vi "all_stages.vi"() -> ()   [LabVIEW 2024]
uses:
  O:/DSG/Tyler/EIC/DIRC/daq/automated/Thorlabs.MotionControl.Controls.dll
  Thorlabs.MotionControl.Controls.dll
  O:/DSG/Tyler/EIC/DIRC/daq/automated/Thorlabs.MotionControl.IntegratedStepperMotorsCLI.dll
  Thorlabs.MotionControl.IntegratedStepperMotorsCLI.dll
  O:/DSG/Tyler/EIC/DIRC/daq/automated/Thorlabs.MotionControl.Benchtop.StepperMotorCLI.dll
  Thorlabs.MotionControl.Benchtop.StepperMotorCLI.dll
  <instrlib>/Keithley 6517/Keithley 6517.lvlib
panel:
  out "ySeq_hist":dbl[][](array[numeric])
  out "xSeq_hist":dbl[][](array[numeric])
  out "xSeq_diff":dbl[](array[numeric])
  out "ySeq_diff":dbl[](array[numeric])
  out "ySeq_in":dbl[](array[numeric])
  out "xSeq_in":dbl[](array[numeric])
  out "ySeq_res":dbl[](array[numeric])
  out "xSeq_res":dbl[](array[numeric])
  in  "go_seq_test":bool
  out "PD Values":cluster{"PD1":dbl, "PD2":dbl, "PD3":dbl}
  out "last-PD":dbl[](array[numeric])=[1.0, 1.0, 1.0]
  in  "move-bar":bool
  in  "mode-select":enum32{"IR", "Pure", "Bulk", "Bar Out"}(radio) caption="Mode Select"
  in  "auto-align-grid":bool
  in  "auto-delta":dbl=0.5
  out "max value":dbl
  out "xOut":dbl
  out "yOut":dbl
  out "max indexes":i32[](array[numeric])
  in  "k":dbl=25.0
  in  "N trials":dbl=16.0
  in  "auto-align":bool
  out "pd_angle":dbl
  out "brewster_angle":dbl
  out "meter-visa":refnum<visa-resource-name>
  out "loop-rate":u32
  out "meter-stat":bool caption="Log Status"
  out "file-stat":bool caption="Log Status"
  out "stage-stat":bool caption="Log Status"
  out "last-save-time":string caption="Time of Last Save:"
  out "pd_y_pos":dbl
  out "pd_x_pos":dbl
  out "bar_y_pos":dbl
  out "bar_x_pos":dbl
  in  "nSamples":dbl=50.0 caption="# Samples"
  out "Current Time:":string
  in  "save-data":bool
  in  "bar-note":bool
  out "pd3_v":dbl caption="PD 3" format="%#.4g"
  out "pd2_v":dbl caption="PD 2" format="%#.4g"
  out "pd1_v":dbl caption="PD 1" format="%#.4g"
  out "meter-error":errorcluster
  out "log-error":errorcluster
  out "log-path":path caption="Path Data Will Save To:"
  out "start-msg":string
  out "stage-error":errorcluster
  in  "PD Angle":refnum<k24>(container)
  in  "Brewster":refnum<k24>(container)
  in  "PD Y":refnum<k24>(container)
  in  "PD X":refnum<k24>(container)
  in  "BAR Y":refnum<k24>(container)
  in  "stop":bool
  in  "BAR X":refnum<k24>(container)
  out "pd-plt":cluster{"[0]":dbl, "[1]":dbl, "[2]":dbl}(graph) caption="Measurement History"
  # "EXPERT DEBUGGING INFO"
  # "A"
  # "A"
  # "A"
  # "Work In Progress - please do not use"
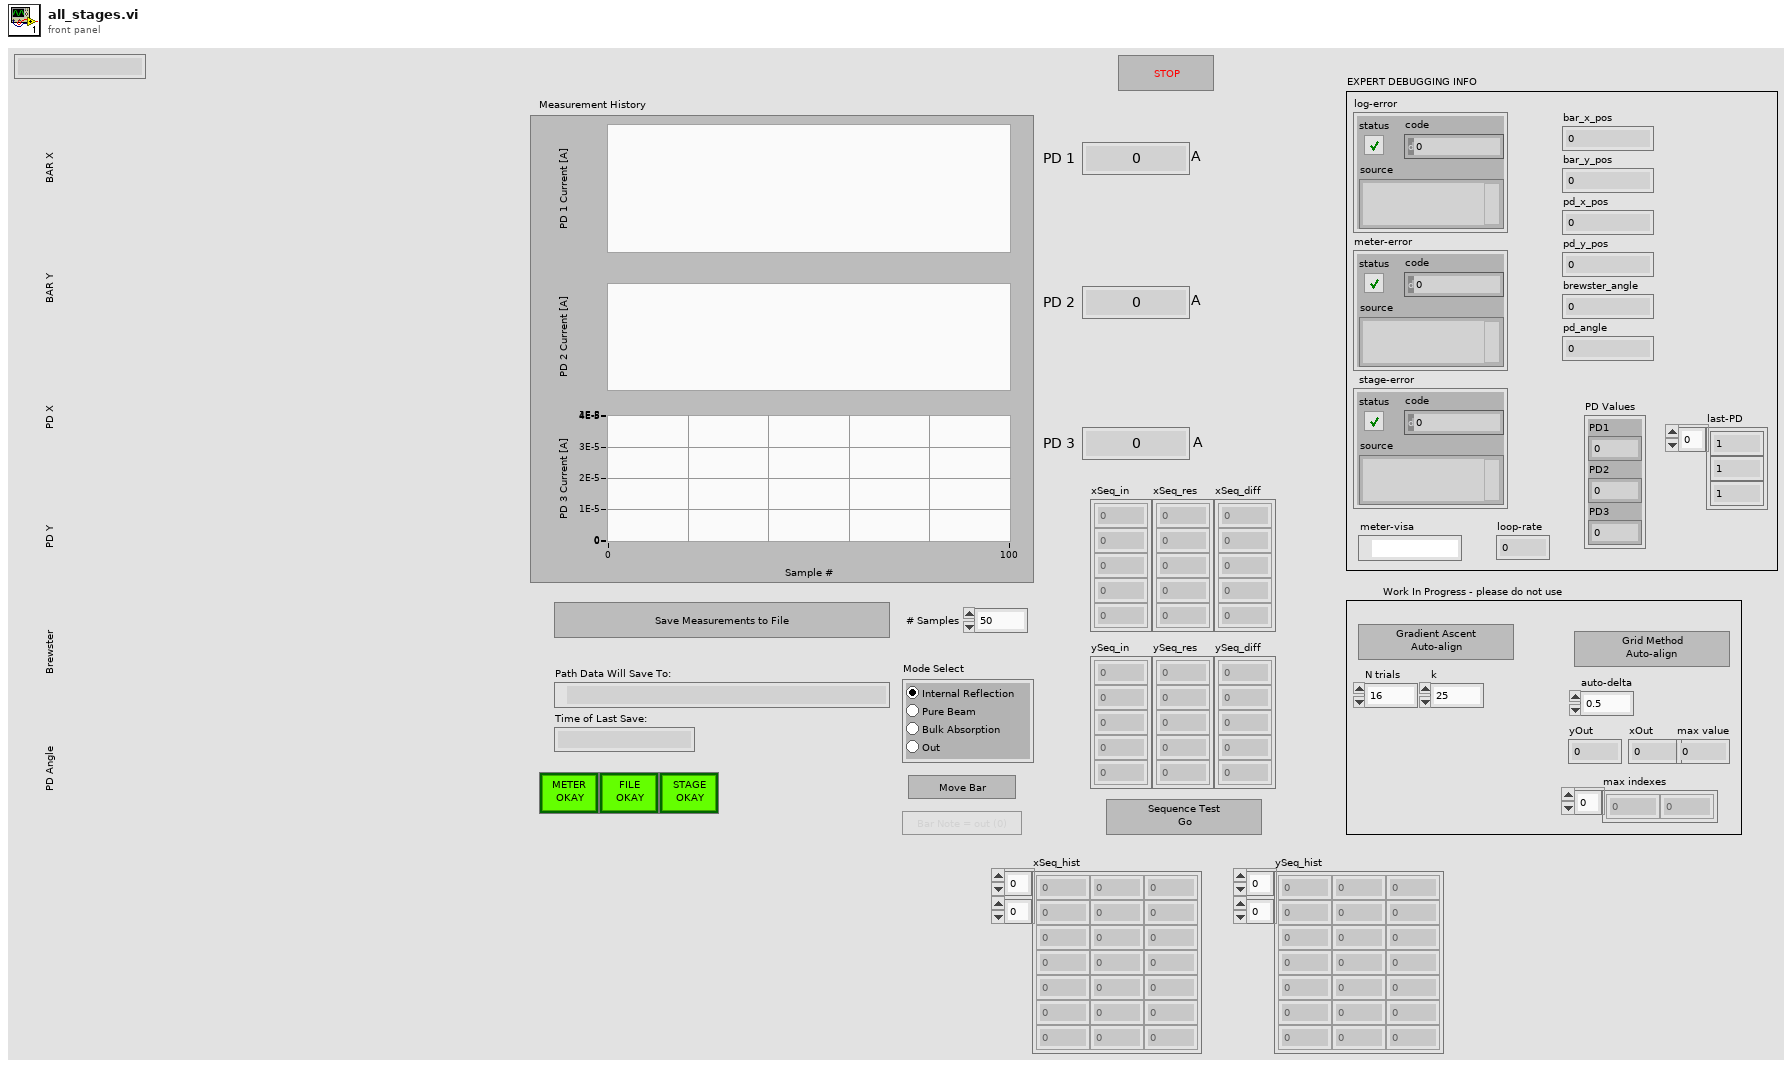
[diagram p1: front panel]
types:
  T1 = cluster{"Bar X":refnum<k24>, "Bar Y":refnum<k24>, "PD X":refnum<k24>, "PD Y":refnum<k24>, "Brewster":refnum<k24>, "PD Angle":refnum<k24>}
  T2 = enum16{"open", "replace", "create", "open or create", "replace or create", "replace or create with confirmation"}
  T3 = cluster{"error":bool, "code":i32, "source":string}
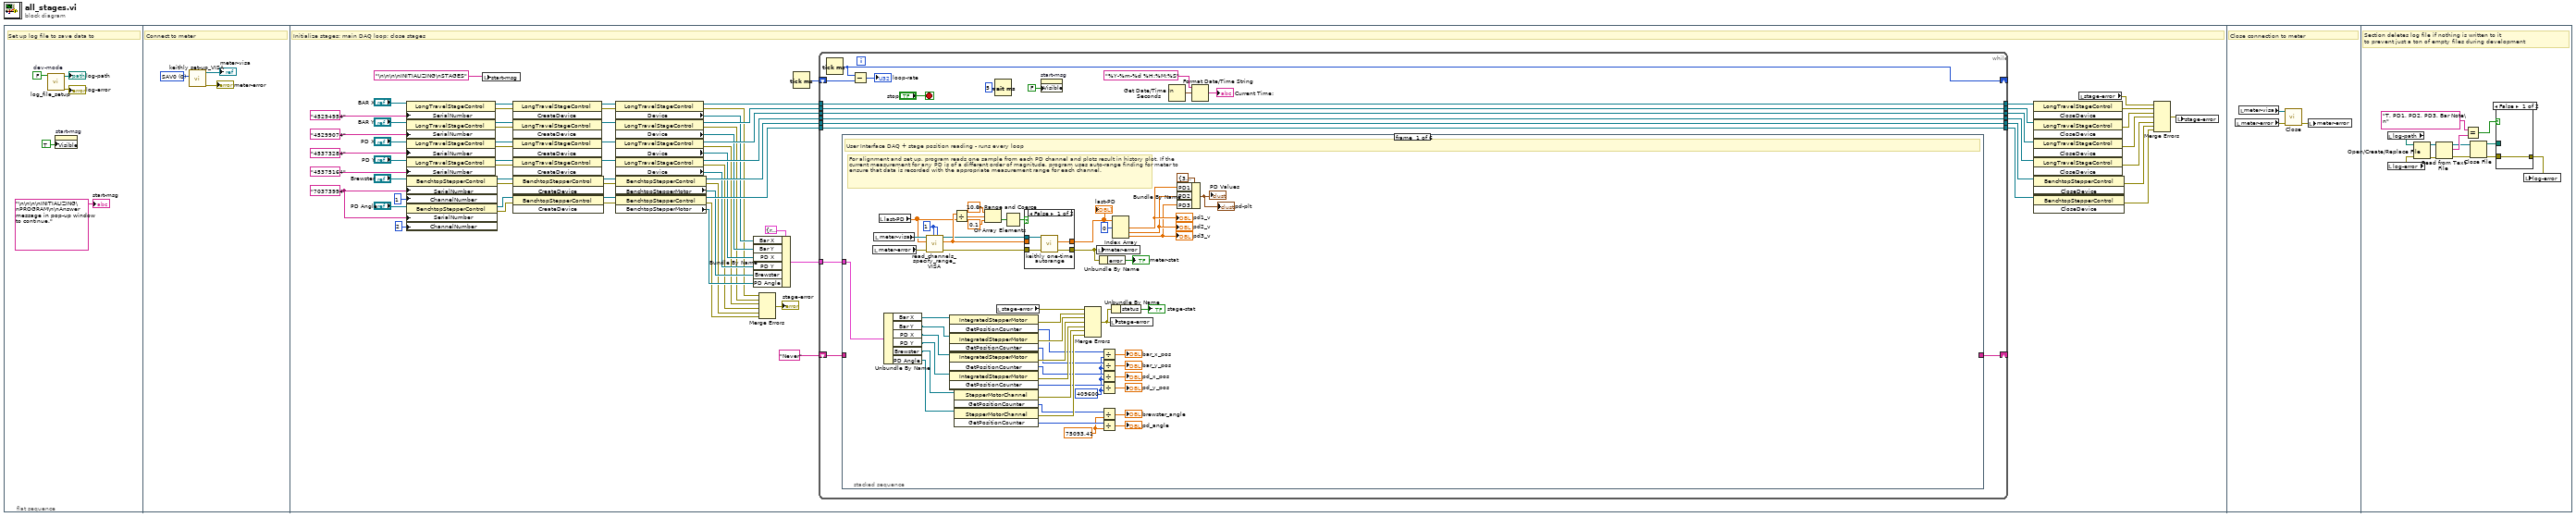
[diagram p0: block diagram]
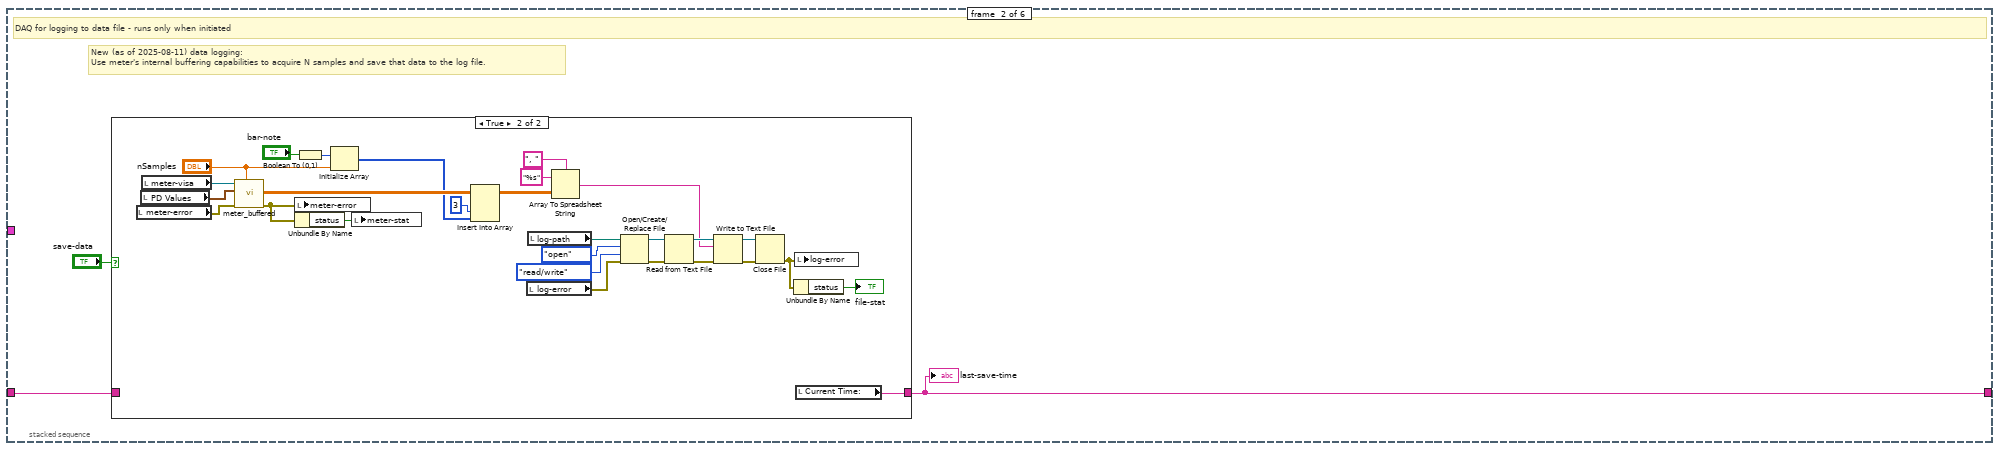
[diagram p3: hidden frame]
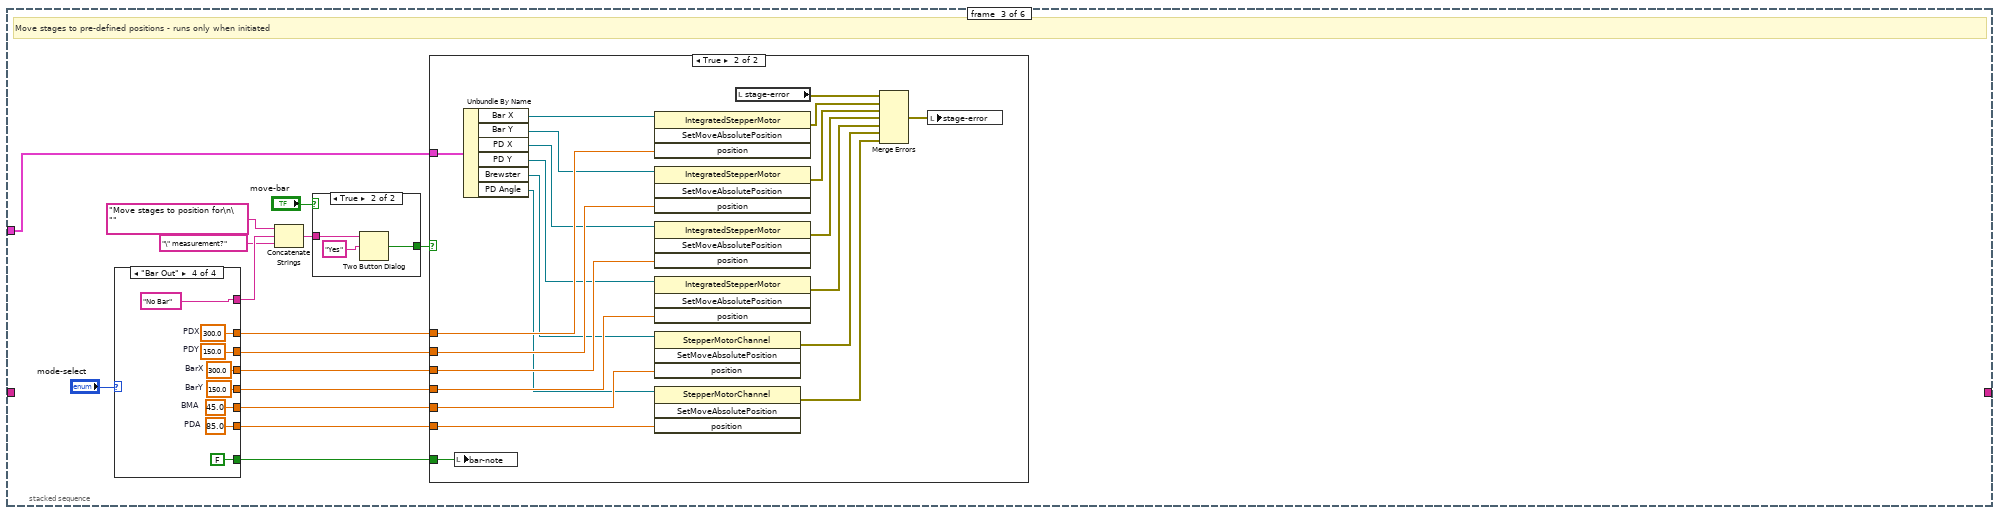
[diagram p5: hidden frame]
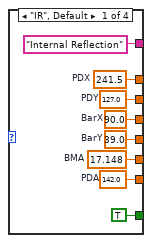
[diagram p7: hidden frame]
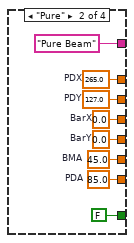
[diagram p8: hidden frame]
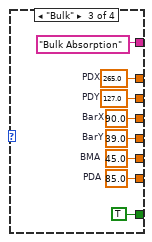
[diagram p9: hidden frame]
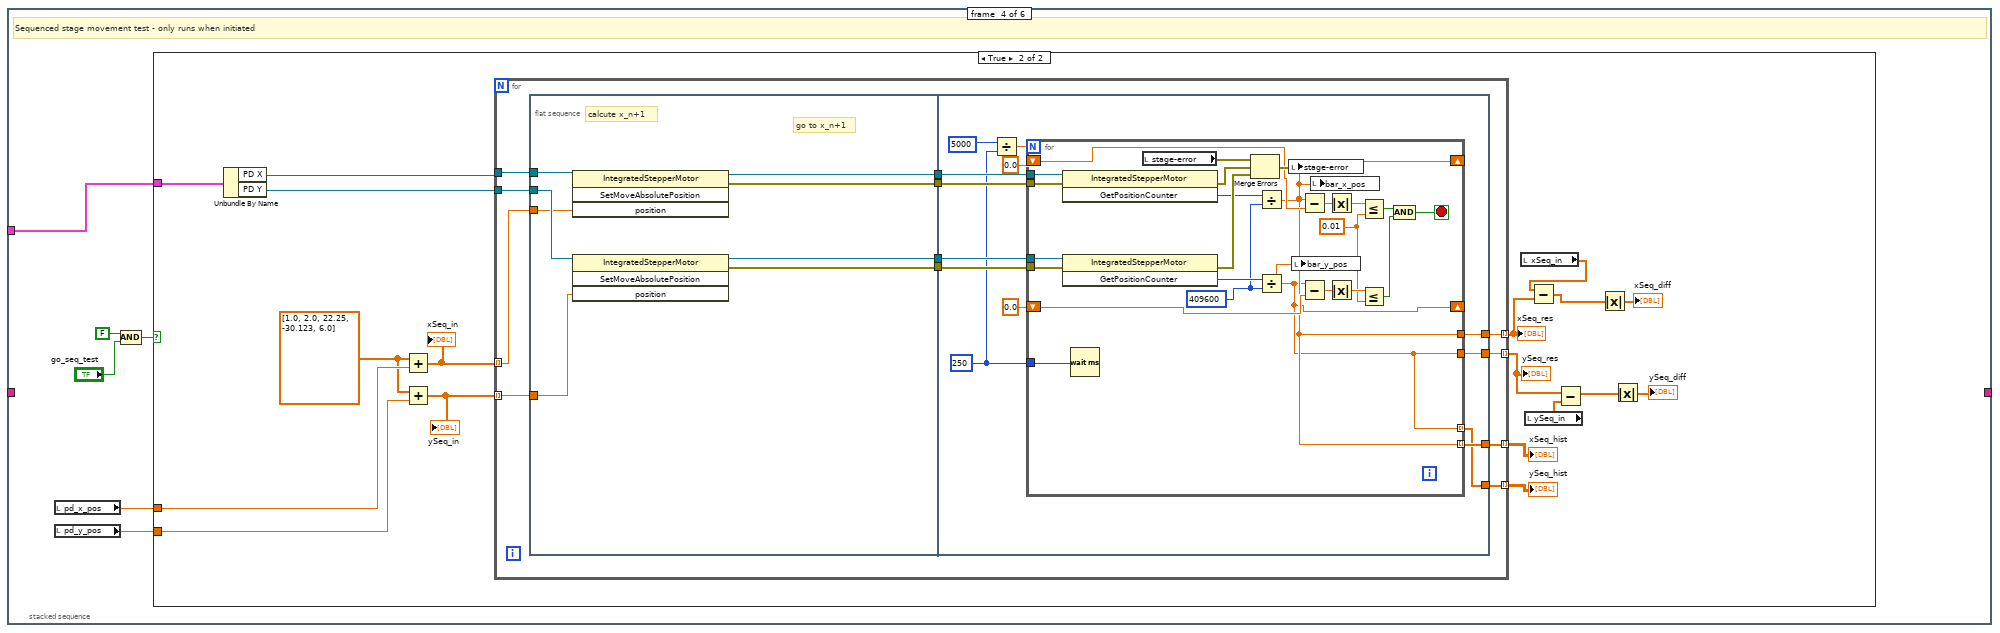
[diagram p11: hidden frame]
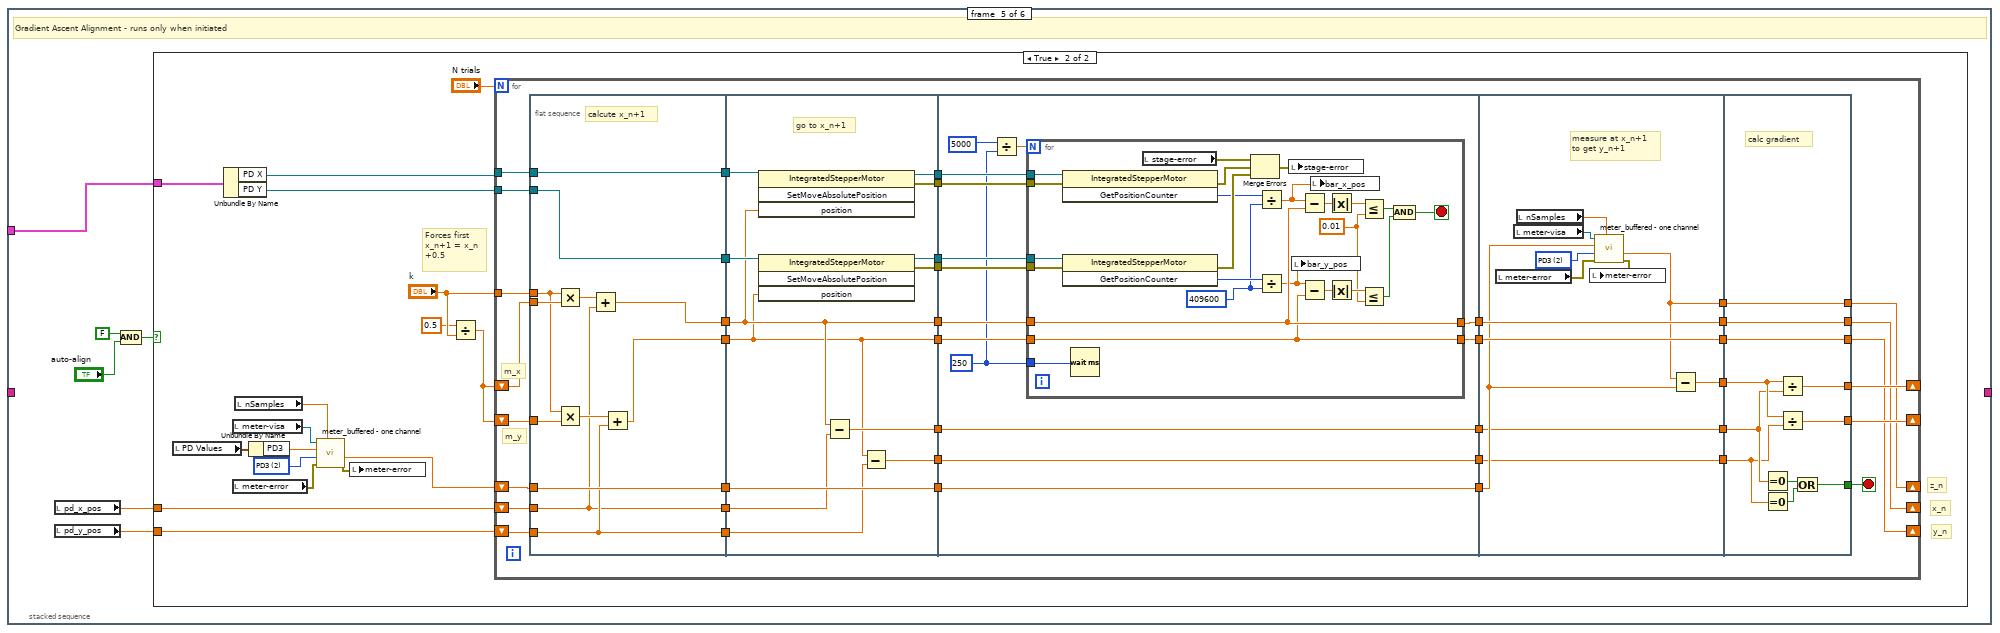
[diagram p13: hidden frame]
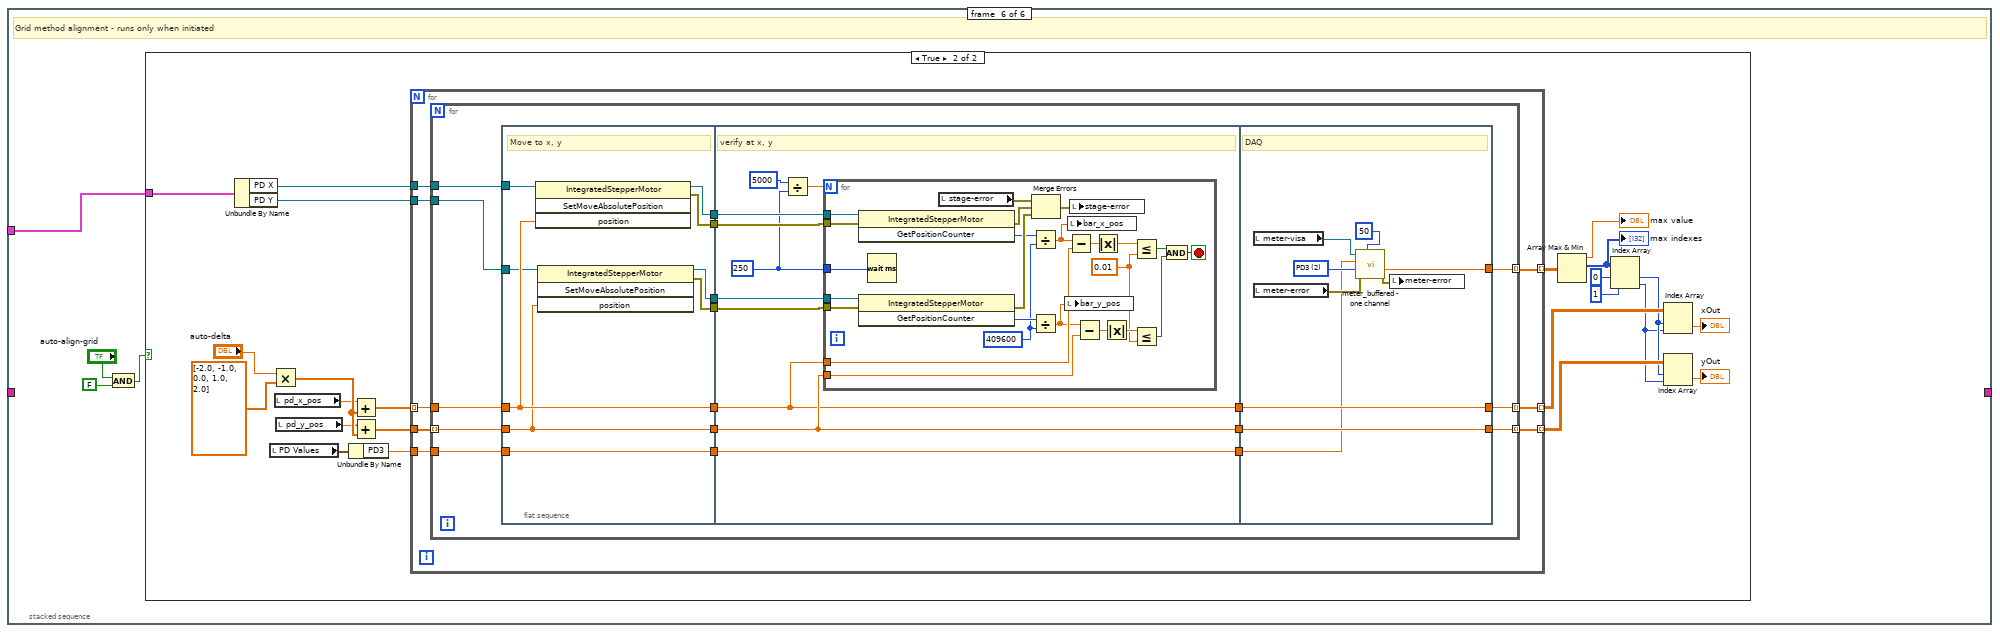
[diagram p15: hidden frame]
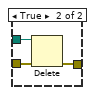
[diagram p17: hidden frame]
diagram:
  n1 = flat-sequence {
    frame #0 {
      w5 = FALSE  # dev-mode
      # "Set up log file to save data to"
      n2 = call "log_file_setup.vi"("dev-mode"=w5) -> ("error out"=→"log-error":errorcluster, "appended path"=→"log-path":path)  [unwired: 8 in, 1 out]
      n3 = property on="start-msg" class="Str"("Visible"=TRUE) -> ()  [unwired: 2 in, 2 out]
      "start-msg" <- "\n\n\n\nINITIALIZING\nPROGRAM\n\nAnswer message in pop-up window to continue." ("String")
    }
    frame #1 {
      w6 = i16 0 items=["SAV0", "SAV1", "SAV2", "SAV3", "SAV4", "SAV5", "SAV6", "SAV7", "SAV8", "SAV9", "RST", "Preset"] ("ConfigOpt")
      # "Connect to meter"
      n4 = call "keithly set-up_VISA.vi"("ConfigOpt"=w6) -> ("error out"=→"meter-error":errorcluster, "meter-VISA"=→"meter-visa":refnum<visa-resource-name>)  [unwired: 9 in]
    }
    frame #2 {
      w57 = "70373994" ("SerialNumber")
      # "Initialize stages; main DAQ loop; close stages"
      n5 = property class="LongTravelStageControl"(reference="BAR X", "SerialNumber"="45294954") -> (reference out=w79:refnum<k24>, error out=w71:errorcluster)  [unwired: 1 in]
      n6 = property class="LongTravelStageControl"(reference="BAR Y", "SerialNumber"="45299074") -> (reference out=w77:refnum<k24>, error out=w70:errorcluster)  [unwired: 1 in]
      n7 = property class="LongTravelStageControl"(reference="PD X", "SerialNumber"="45373284") -> (reference out=w74:refnum<k24>, error out=w69:errorcluster)  [unwired: 1 in]
      n8 = property class="LongTravelStageControl"(reference="PD Y", "SerialNumber"="45375164") -> (reference out=w73:refnum<k24>, error out=w68:errorcluster)  [unwired: 1 in]
      n9 = property class="BenchtopStepperControl"(reference="Brewster", "SerialNumber"=w57, "ChannelNumber"=1) -> (reference out=w26:refnum<k24>, error out=w25:errorcluster)  [unwired: 1 in]
      n10 = property class="BenchtopStepperControl"(reference="PD Angle", "SerialNumber"=w57, "ChannelNumber"=2) -> (reference out=w27:refnum<k24>, error out=w24:errorcluster)  [unwired: 1 in]
      n11 = local write "start-msg"("\n\n\n\nINITIALIZING\nSTAGES" ("String")) -> ()
      n12 = invoke class="LongTravelStageControl" method="CreateDevice"(reference=w79, error in=w71) -> (reference out=w49:refnum<k24>, error out=w45:errorcluster)  [unwired: 1 in, 1 out]
      n13 = invoke class="LongTravelStageControl" method="CreateDevice"(reference=w77, error in=w70) -> (reference out=w48:refnum<k24>)  [unwired: 1 in, 2 out]
      n14 = invoke class="LongTravelStageControl" method="CreateDevice"(reference=w74, error in=w69) -> (reference out=w47:refnum<k24>)  [unwired: 1 in, 2 out]
      n15 = invoke class="LongTravelStageControl" method="CreateDevice"(reference=w73, error in=w68) -> (reference out=w46:refnum<k24>)  [unwired: 1 in, 2 out]
      n16 = invoke class="BenchtopStepperControl" method="CreateDevice"(reference=w26, error in=w25) -> (reference out=w38:refnum<k24>, error out=w40:errorcluster)  [unwired: 1 in, 1 out]
      n17 = invoke class="BenchtopStepperControl" method="CreateDevice"(reference=w27, error in=w24) -> (reference out=w39:refnum<k24>, error out=w37:errorcluster)  [unwired: 1 in, 1 out]
      n18 = property class="LongTravelStageControl"(reference=w49, error in=w45) -> (reference out=w44:refnum<k24>, error out=w10:errorcluster, "Device"=w22:refnum<k24>)
      n19 = property class="LongTravelStageControl"(reference=w48) -> (reference out=w43:refnum<k24>, error out=w15:errorcluster, "Device"=w21:refnum<k24>)  [unwired: 1 in]
      n20 = property class="LongTravelStageControl"(reference=w47) -> (reference out=w42:refnum<k24>, error out=w14:errorcluster, "Device"=w20:refnum<k24>)  [unwired: 1 in]
      n21 = property class="LongTravelStageControl"(reference=w46) -> (reference out=w41:refnum<k24>, error out=w13:errorcluster, "Device"=w19:refnum<k24>)  [unwired: 1 in]
      n22 = property class="BenchtopStepperControl"(reference=w38, error in=w40) -> (reference out=w35:refnum<k24>, error out=w12:errorcluster, "BenchtopStepperMotor"=w18:refnum<k24>)
      n23 = property class="BenchtopStepperControl"(reference=w39, error in=w37) -> (reference out=w36:refnum<k24>, error out=w11:errorcluster, "BenchtopStepperMotor"=w16:refnum<k24>)
      n24 = Bundle By Name(cluster=T1 {"Bar X"=refnum, "Bar Y"=refnum, "PD X"=refnum, "PD Y"=refnum, "Brewster"=refnum, "PD Angle"=refnum}, "Bar X"=w22, "Bar Y"=w21, "PD X"=w20, "PD Y"=w19, "Brewster"=w18, "PD Angle"=w16) -> (w17:T1)
      n25 = Merge Errors(w10, w15, w14, w13, w12, w11) -> (→"stage-error":errorcluster)
      n26 = Tick Count (ms)() -> (millisecond timer value=w31:u32)
      n27 = while {
        tunnel: w44 -> [w97]
        tunnel: [w97] -> w78
        tunnel: w41 -> [w94]
        tunnel: w42 -> [w95]
        tunnel: w43 -> [w96]
        tunnel: [w96] -> w65
        tunnel: [w95] -> w66
        tunnel: [w94] -> w67
        tunnel: w35 -> [w93]
        tunnel: [w93] -> w59
        tunnel: w36 -> [w92]
        tunnel: [w92] -> w56
        shift-right: [w85] -> _
        shift-left: "Never" ("date/time string") -> [w90]
        shift-right: [w89] -> _
        shift-left: w31 -> [w88]
        tunnel: w17 -> [w86]
        stop <- "stop" stop-if-true
        n28 = Tick Count (ms)() -> (millisecond timer value=w89:u32)
        n29 = stacked-sequence {
          tunnel: [_ w157 _ _ _ _] -> w85
          tunnel: w90 -> [_ w158 _ _ _ _]
          tunnel: w86 -> [w141 _ w188 w264 w345 w495]
          frame #0 {
            w111 = u32 1 ("preDAQ  wait ms")
            w120 = 75093.41 ("GetPositionCounter")
            w121 = 409600 ("y")
            # "For alignment and set up, program reads one sample from each PD channel and plots result in history plot. If the current measurement for any PD is of a different order of magnitude, program uses auto-range finding for meter to ensure that data is recorded with the appropriate measurement range for each channel."
            # "User Interface DAQ + stage position reading - runs every loop"
            n30 = local read "meter-error"() -> (w112:errorcluster)
            n31 = local read "meter-visa"() -> (w113:refnum<visa-resource-name>)
            n32 = local read "last-PD"() -> (w102:dbl[])
            n33 = Unbundle By Name(w141) -> ("Bar X"=w140:refnum<k24>, "Bar Y"=w139:refnum<k24>, "PD X"=w138:refnum<k24>, "PD Y"=w137:refnum<k24>, "Brewster"=w136:refnum<k24>, "PD Angle"=w135:refnum<k24>)
            n34 = call "read_channels_specify_range_VISA.vi"("postDAQ  wait ms"=w111, "preDAQ  wait ms"=w111, "error in"=w112, "range"=w102, "VISA resource in"=w113) -> ("error out"=w105:T3, "data"=w104:dbl[], "VISA resource out"=w103:refnum<visa-resource-name>)  [unwired: 4 in]
            n35 = invoke class="IntegratedStepperMotor" method="GetPositionCounter"(reference=w140) -> (error out=w133:errorcluster, "GetPositionCounter"=w127:i32)  [unwired: 2 in, 1 out]
            n36 = invoke class="IntegratedStepperMotor" method="GetPositionCounter"(reference=w139) -> (error out=w132:errorcluster, "GetPositionCounter"=w126:i32)  [unwired: 2 in, 1 out]
            n37 = invoke class="IntegratedStepperMotor" method="GetPositionCounter"(reference=w138) -> (error out=w131:errorcluster, "GetPositionCounter"=w125:i32)  [unwired: 2 in, 1 out]
            n38 = invoke class="IntegratedStepperMotor" method="GetPositionCounter"(reference=w137) -> (error out=w130:errorcluster, "GetPositionCounter"=w124:i32)  [unwired: 2 in, 1 out]
            n39 = Divide(x=w104, y=w102) -> (x/y=w108:dbl[])
            n40 = invoke class="StepperMotorChannel" method="GetPositionCounter"(reference=w136) -> (error out=w129:errorcluster, "GetPositionCounter"=w123:i32)  [unwired: 2 in, 1 out]
            n41 = invoke class="StepperMotorChannel" method="GetPositionCounter"(reference=w135) -> (error out=w128:errorcluster, "GetPositionCounter"=w122:i32)  [unwired: 2 in, 1 out]
            n42 = In Range and Coerce(upper limit=10.0, x=w108, lower limit=0.1) -> (In Range?=w106:bool[])  [unwired: 1 out]
            n43 = local read "stage-error"() -> (w134:errorcluster)
            n44 = Or Array Elements(Boolean array=w106) -> (logical OR=w107:bool)
            n45 = case shown="False" w107 {
              tunnel: w105 -> [w153 w155]
              tunnel: [w152 w155] -> w147
              tunnel: [w151 w154] -> w142
              tunnel: w104 -> [_ w154]
              tunnel: w103 -> [w150 _]
              frame False {
                n46 = call "keithly one-time autorange.vi"("error in"=w153, "VISA in"=w150) -> ("error out"=w152:errorcluster, "data"=w151:dbl[])  [unwired: 7 in, 1 out]
              }
              frame True {
              }
            }
            "last-PD" <- w142
            n47 = Merge Errors(w134, w133, w132, w131, w130, w129, w128) -> (w99:errorcluster)
            n48 = local write "meter-error"(w147) -> ()
            n49 = Unbundle By Name(w147) -> ("error"=→"meter-stat":bool)
            n50 = Divide(x=w127, y=w121) -> (x/y=→"bar_x_pos":dbl)
            n51 = Divide(x=w126, y=w121) -> (x/y=→"bar_y_pos":dbl)
            n52 = Divide(x=w125, y=w121) -> (x/y=→"pd_x_pos":dbl)
            n53 = Divide(x=w124, y=w121) -> (x/y=→"pd_y_pos":dbl)
            n54 = Divide(x=w123, y=w120) -> (x/y=→"brewster_angle":dbl)
            n55 = Divide(x=w122, y=w120) -> (x/y=→"pd_angle":dbl)
            n56 = local write "stage-error"(w99) -> ()
            n57 = Unbundle By Name(w99) -> ("status"=→"stage-stat":bool)
            n58 = Index Array(array=w142, index #1=0 ("index")) -> (element #1=w145:dbl, element #2=w144:dbl, element #3=w143:dbl)  [unwired: 2 in]
            "pd3_v" <- w143
            "pd2_v" <- w144
            "pd1_v" <- w145
            n59 = Bundle By Name(cluster=cluster{"PD1":dbl, "PD2":dbl, "PD3":dbl} {"PD1"=3e-05, "PD2"=3e-05, "PD3"=3e-05} ("PD ranges"), "PD1"=w145, "PD2"=w144, "PD3"=w143) -> (→"pd-plt" →"PD Values":cluster{"PD1":dbl, "PD2":dbl, "PD3":dbl})
          }
          frame #1 {
            # "New (as of 2025-08-11) data logging:\nUse meter's internal buffering capabilities to acquire N samples and save that data to the log file."
            # "DAQ for logging to data file - runs only when initiated"
            n60 = case shown="True" "save-data" {
              tunnel: w158 -> [w159 _]
              tunnel: [w159 w166] -> w157
              frame False {
              }
              frame True {
                n61 = local read "meter-error"() -> (w186:errorcluster)
                n62 = local read "PD Values"() -> (w160:cluster{"PD1":dbl, "PD2":dbl, "PD3":dbl})
                n63 = local read "meter-visa"() -> (w187:refnum<visa-resource-name>)
                n64 = call "meter_buffered.vi"("Samples"="nSamples", "error in"=w186, "PD ranges"=w160, "meter-VISA"=w187) -> ("error out"=w161:errorcluster, "ch1-3 data"=w174:dbl[][])  [unwired: 5 in, 1 out]
                n65 = local write "meter-error"(w161) -> ()
                n66 = Unbundle By Name(w161) -> ("status"=w162:bool)
                n67 = Boolean To (0,1)(Boolean="bar-note") -> (0, 1=w171:i16)
                n68 = Initialize Array(w171, "nSamples") -> (w172:i16[])
                n69 = local write "meter-stat"(w162) -> ()
                n70 = Insert Into Array(array=w174, index (col)=3 ("disabled index (col)"), new element=w172) -> (w168:dbl[][])  [unwired: 1 in]
                n71 = local read "log-error"() -> (w184:errorcluster)
                n72 = local read "log-path"() -> (w185:path)
                n73 = Array To Spreadsheet String(delimiter (Tab)=", ", array=w168, 3:"%s" ("format string")) -> (spreadsheet string=w167:string)
                n74 = Open/Create/Replace File(file path (use dialog)=w185, error in=w184, operation (0:open)=T2."open", access (0:read/write)=enum16{"read/write", "read-only", "write-only"}."read/write") -> (refnum out=w183:refnum<file>, error out=w179:errorcluster)  [unwired: 2 in, 1 out]
                n75 = Read from Text File(file (use dialog)=w183, error in=w179) -> (refnum out=w180:refnum<file>, error out=w178:errorcluster)  [unwired: 2 in, 2 out]
                n76 = Write to Text File(file (use dialog)=w180, text=w167, error in=w178) -> (refnum out=w182:refnum<file>, error out=w181:errorcluster)  [unwired: 1 in, 1 out]
                n77 = Close File(refnum=w182, error in=w181) -> (error out=w177:errorcluster)  [unwired: 1 out]
                n78 = Unbundle By Name(w177) -> ("status"=→"file-stat":bool)
                n79 = local write "log-error"(w177) -> ()
                n80 = local read "Current Time:"() -> (w166:string)
              }
            }
            "last-save-time" <- w157
          }
          frame #2 {
            # "Move stages to pre-defined positions - runs only when initiated"
            n81 = case shown="\"Bar Out\"" "mode-select" {
              tunnel: [w214 w222 w230 w238] -> w201
              tunnel: [w209 w221 w229 w237] -> w200
              tunnel: [w210 w220 w228 w236] -> w199
              tunnel: [w211 w219 w227 w235] -> w198
              tunnel: [w212 w218 w226 w234] -> w197
              tunnel: [w213 w217 w225 w233] -> w196
              tunnel: [TRUE FALSE TRUE FALSE] -> w195
              tunnel: ["Internal Reflection" "Pure Beam" "Bulk Absorption" "No Bar"] -> w192
              frame "IR", Default {
                w213 = 142.0  # PDA
                w209 = 127.0  # PDY
                w214 = 241.5  # PDX
                w211 = 39.0  # BarY
                w210 = 90.0  # BarX
                w212 = 17.148  # BMA
              }
              frame "Pure" {
                w217 = 85.0  # PDA
                w221 = 127.0  # PDY
                w222 = 265.0  # PDX
                w219 = 0.0  # BarY
                w220 = 0.0  # BarX
                w218 = 45.0  # BMA
              }
              frame "Bulk" {
                w225 = 85.0  # PDA
                w229 = 127.0  # PDY
                w230 = 265.0  # PDX
                w227 = 39.0  # BarY
                w228 = 90.0  # BarX
                w226 = 45.0  # BMA
              }
              frame "Bar Out" {
                w233 = 85.0  # PDA
                w237 = 150.0  # PDY
                w238 = 300.0  # PDX
                w235 = 150.0  # BarY
                w236 = 300.0  # BarX
                w234 = 45.0  # BMA
              }
            }
            n82 = Concatenate Strings("Move stages to position for\n\"", w192, "\" measurement?" ("string")) -> (w190:string)
            n83 = case shown="True" "move-bar" {
              selector: "move-bar" -> [w203 _]
              tunnel: [w203 w205] -> w193
              tunnel: w190 -> [_ w204]
              frame False {
              }
              frame True {
                n84 = Two Button Dialog(message=w204, 2:"Yes" ("T button name (\"OK\")")) -> (T button?=w205:bool)  [unwired: 1 in]
              }
            }
            n85 = case shown="True" w193 {
              tunnel: w201 -> [_ w252]
              tunnel: w200 -> [_ w251]
              tunnel: w199 -> [_ w250]
              tunnel: w198 -> [_ w249]
              tunnel: w197 -> [_ w248]
              tunnel: w196 -> [_ w247]
              tunnel: w195 -> [_ w246]
              tunnel: w188 -> [_ w245]
              frame False {
              }
              frame True {
                n86 = local write "bar-note"(w246) -> ()
                n87 = Unbundle By Name(w245) -> ("Bar X"=w244:refnum<k24>, "Bar Y"=w239:refnum<k24>, "PD X"=w240:refnum<k24>, "PD Y"=w241:refnum<k24>, "Brewster"=w242:refnum<k24>, "PD Angle"=w243:refnum<k24>)
                n88 = invoke class="IntegratedStepperMotor" method="SetMoveAbsolutePosition"(reference=w244, "position"=w252) -> (error out=w259:errorcluster)  [unwired: 2 in, 3 out]
                n89 = invoke class="IntegratedStepperMotor" method="SetMoveAbsolutePosition"(reference=w239, "position"=w251) -> (error out=w258:errorcluster)  [unwired: 2 in, 3 out]
                n90 = invoke class="IntegratedStepperMotor" method="SetMoveAbsolutePosition"(reference=w240, "position"=w250) -> (error out=w257:errorcluster)  [unwired: 2 in, 3 out]
                n91 = invoke class="IntegratedStepperMotor" method="SetMoveAbsolutePosition"(reference=w241, "position"=w249) -> (error out=w256:errorcluster)  [unwired: 2 in, 3 out]
                n92 = invoke class="StepperMotorChannel" method="SetMoveAbsolutePosition"(reference=w242, "position"=w248) -> (error out=w255:errorcluster)  [unwired: 2 in, 3 out]
                n93 = invoke class="StepperMotorChannel" method="SetMoveAbsolutePosition"(reference=w243, "position"=w247) -> (error out=w254:errorcluster)  [unwired: 2 in, 3 out]
                n94 = local read "stage-error"() -> (w260:errorcluster)
                n95 = Merge Errors(w260, w259, w258, w257, w256, w255, w254) -> (w253:errorcluster)
                n96 = local write "stage-error"(w253) -> ()
              }
            }
          }
          frame #3 {
            # "Sequenced stage movement test - only runs when initiated"
            n97 = local read "pd_x_pos"() -> (w266:dbl)
            n98 = local read "pd_y_pos"() -> (w265:dbl)
            n99 = And(x=FALSE, y="go_seq_test") -> (x .and. y?=w263:bool)
            n100 = case shown="True" w263 {
              tunnel: w266 -> [_ w280]
              tunnel: w265 -> [_ w278]
              tunnel: w264 -> [_ w284]
              frame False {
              }
              frame True {
                w279 = dbl[] [1.0, 2.0, 22.25, -30.123, 6.0]
                n101 = Unbundle By Name(w284) -> ("PD X"=w283:refnum<k24>, "PD Y"=w282:refnum<k24>)
                n102 = Add(x=w279, y=w280) -> (x+y=w281:dbl[])
                "xSeq_in" <- w281
                n103 = Add(x=w279, y=w278) -> (x+y=w277:dbl[])
                "ySeq_in" <- w277
                n104 = for {
                  tunnel: w283 -> [w292]
                  tunnel: w282 -> [w291]
                  tunnel: w281 -> [w290] mode=indexing
                  tunnel: w277 -> [w289] mode=indexing
                  tunnel: [w288] -> w276 mode=indexing
                  tunnel: [w287] -> w273 mode=indexing
                  tunnel: [w286] -> w268 mode=indexing
                  tunnel: [w285] -> w267 mode=indexing
                  n105 = flat-sequence {
                    tunnel: [w304] -> w296
                    tunnel: [w303] -> w295
                    tunnel: [w302] -> w294
                    tunnel: [w301] -> w293
                    tunnel: w291 -> [w299]
                    tunnel: w292 -> [w300]
                    tunnel: w290 -> [w298]
                    tunnel: w289 -> [w297]
                    tunnel: w293 -> [w314]
                    tunnel: w294 -> [w315]
                    tunnel: w295 -> [w316]
                    tunnel: w296 -> [w317]
                    tunnel: [w310] -> w288
                    tunnel: [w309] -> w287
                    tunnel: [w306] -> w286
                    tunnel: [w305] -> w285
                    frame #0 {
                      # "calcute x_n+1"
                      # "go to x_n+1"
                      n106 = invoke class="IntegratedStepperMotor" method="SetMoveAbsolutePosition"(reference=w300, "position"=w298) -> (reference out=w304:refnum<k24>, error out=w302:errorcluster)  [unwired: 2 in, 2 out]
                      n107 = invoke class="IntegratedStepperMotor" method="SetMoveAbsolutePosition"(reference=w299, "position"=w297) -> (reference out=w303:refnum<k24>, error out=w301:errorcluster)  [unwired: 2 in, 2 out]
                    }
                    frame #1 {
                      w311 = 250
                      n108 = Divide(x=5000, y=w311) -> (x/y=w313:dbl)
                      n109 = for {
                        N: w313 -> [_]
                        tunnel: w317 -> [w341]
                        tunnel: w316 -> [w340]
                        tunnel: w315 -> [w339]
                        tunnel: w314 -> [w338]
                        tunnel: w311 -> [w322]
                        tunnel: [w319] -> w310
                        tunnel: [w318] -> w309
                        shift-right: [w319] -> _
                        shift-left: 0.0 -> [w321]
                        shift-right: [w318] -> _
                        shift-left: 0.0 -> [w320]
                        tunnel: [w319] -> w306 mode=indexing
                        tunnel: [w318] -> w305 mode=indexing
                        stop <- w323 stop-if-true
                        w326 = 0.01 ("y")
                        w331 = 409600 ("y")
                        n110 = invoke class="IntegratedStepperMotor" method="GetPositionCounter"(reference=w341, error in=w339) -> (error out=w335:errorcluster, "GetPositionCounter"=w333:i32)  [unwired: 1 in, 1 out]
                        n111 = invoke class="IntegratedStepperMotor" method="GetPositionCounter"(reference=w340, error in=w338) -> (error out=w334:errorcluster, "GetPositionCounter"=w332:i32)  [unwired: 1 in, 1 out]
                        n112 = Wait (ms)(milliseconds to wait=w322) -> ()  [unwired: 1 out]
                        n113 = local read "stage-error"() -> (w337:errorcluster)
                        n114 = Merge Errors(w337, w335, w334) -> (w336:errorcluster)
                        n115 = Divide(x=w333, y=w331) -> (x/y=w319:dbl)
                        n116 = Divide(x=w332, y=w331) -> (x/y=w318:dbl)
                        n117 = local write "stage-error"(w336) -> ()
                        n118 = local write "bar_y_pos"(w318) -> ()
                        n119 = Subtract(x=w319, y=w321) -> (x-y=w330:dbl)
                        n120 = Subtract(x=w318, y=w320) -> (x-y=w329:dbl)
                        n121 = local write "bar_x_pos"(w319) -> ()
                        n122 = Absolute Value(x=w330) -> (abs(x)=w328:dbl)
                        n123 = Absolute Value(x=w329) -> (abs(x)=w327:dbl)
                        n124 = Less Or Equal?(x=w328, y=w326) -> (x <= y?=w325:bool)
                        n125 = Less Or Equal?(x=w327, y=w326) -> (x <= y?=w324:bool)
                        n126 = And(x=w325, y=w324) -> (x .and. y?=w323:bool)
                      }
                    }
                  }
                }
                "xSeq_res" <- w276
                "ySeq_res" <- w273
                "xSeq_hist" <- w268
                "ySeq_hist" <- w267
                n127 = local read "xSeq_in"() -> (w269:dbl[])
                n128 = local read "ySeq_in"() -> (w270:dbl[])
                n129 = Subtract(x=w269, y=w276) -> (x-y=w275:dbl[])
                n130 = Subtract(x=w273, y=w270) -> (x-y=w272:dbl[])
                n131 = Absolute Value(x=w275) -> (abs(x)=→"xSeq_diff":dbl[])
                n132 = Absolute Value(x=w272) -> (abs(x)=→"ySeq_diff":dbl[])
              }
            }
          }
          frame #4 {
            # "Gradient Ascent Alignment - runs only when initiated"
            n133 = local read "pd_x_pos"() -> (w347:dbl)
            n134 = local read "pd_y_pos"() -> (w346:dbl)
            n135 = And(x=FALSE, y="auto-align") -> (x .and. y?=w344:bool)
            n136 = case shown="True" w344 {
              tunnel: w347 -> [_ w359]
              tunnel: w346 -> [_ w360]
              tunnel: w345 -> [_ w350]
              frame False {
              }
              frame True {
                w358 = u16 2 items=["PD1", "PD2", "PD3"] ("Photodiode Select")
                # "y_n"
                # "x_n"
                # "z_n"
                # "Forces first x_n+1 = x_n +0.5"
                n137 = local read "PD Values"() -> (w352:cluster{"PD1":dbl, "PD2":dbl, "PD3":dbl})
                n138 = Unbundle By Name(w350) -> ("PD X"=w349:refnum<k24>, "PD Y"=w348:refnum<k24>)
                n139 = local read "meter-visa"() -> (w355:refnum<visa-resource-name>)
                n140 = local read "meter-error"() -> (w356:errorcluster)
                n141 = local read "nSamples"() -> (w353:dbl)
                n142 = Unbundle By Name(w352) -> ("PD3"=w351:dbl)
                n143 = call "meter_buffered - one channel.vi"("Samples"=w353, "error in"=w356, "Channel"=w358, "PD Range"=w351, "meter-VISA"=w355) -> ("error out"=w357:errorcluster, "avg"=w354:dbl)  [unwired: 3 in, 2 out]
                n144 = local write "meter-error"(w357) -> ()
                n145 = Divide(x=0.5, y="k") -> (x/y=w364:dbl)
                n146 = for {
                  N: "N trials" -> [_]
                  shift-right: [w388] -> _
                  shift-left: w359 -> [w400]
                  shift-right: [w389] -> _
                  shift-left: w354 -> [w401]
                  tunnel: "k" -> [w405]
                  shift-right: [w387] -> _
                  shift-left: w360 -> [w397]
                  shift-right: [w392] -> _
                  shift-left: w364 -> [w390]
                  shift-right: [w393] -> _
                  shift-left: w364 -> [w391]
                  tunnel: w349 -> [w375]
                  tunnel: w348 -> [w373]
                  stop <- w376 stop-if-true
                  # "m_y"
                  # "m_x"
                  n147 = flat-sequence {
                    tunnel: w405 -> [w412]
                    tunnel: [w417] -> w404
                    tunnel: w401 -> [w416]
                    tunnel: [w416] -> w402
                    tunnel: w400 -> [w406]
                    tunnel: [w406] -> w399
                    tunnel: [w408] -> w398
                    tunnel: w397 -> [w408]
                    tunnel: [w415] -> w396
                    tunnel: w391 -> [w414]
                    tunnel: w390 -> [w413]
                    tunnel: w375 -> [w411]
                    tunnel: [w411] -> w374
                    tunnel: w373 -> [w410]
                    tunnel: [w410] -> w372
                    tunnel: w404 -> [w423]
                    tunnel: [w423] -> w386
                    tunnel: w402 -> [w430]
                    tunnel: [w430] -> w384
                    tunnel: w399 -> [w422]
                    tunnel: w398 -> [w420]
                    tunnel: w396 -> [w419]
                    tunnel: [w419] -> w382
                    tunnel: [w429] -> w380
                    tunnel: [w428] -> w379
                    tunnel: [w427] -> w378
                    tunnel: [w426] -> w377
                    tunnel: w374 -> [w425]
                    tunnel: w372 -> [w424]
                    tunnel: [w421] -> w371
                    tunnel: [w418] -> w370
                    tunnel: w386 -> [w438]
                    tunnel: [w437] -> w385
                    tunnel: w384 -> [w444]
                    tunnel: [w444] -> w383
                    tunnel: w382 -> [w439]
                    tunnel: [w436] -> w381
                    tunnel: w380 -> [w443]
                    tunnel: w379 -> [w442]
                    tunnel: w378 -> [w441]
                    tunnel: w377 -> [w440]
                    tunnel: w371 -> [w432]
                    tunnel: w370 -> [w431]
                    tunnel: [w432] -> w368
                    tunnel: [w431] -> w365
                    tunnel: w385 -> [w480]
                    tunnel: [w480] -> w403
                    tunnel: w383 -> [w473]
                    tunnel: w381 -> [w479]
                    tunnel: [w479] -> w395
                    tunnel: [w474] -> w394
                    tunnel: [w472] -> w369
                    tunnel: w368 -> [w471]
                    tunnel: [w471] -> w367
                    tunnel: [w470] -> w366
                    tunnel: w365 -> [w470]
                    tunnel: w403 -> [w489]
                    tunnel: [w489] -> w388
                    tunnel: w395 -> [w488]
                    tunnel: [w488] -> w387
                    tunnel: w394 -> [w487]
                    tunnel: [w487] -> w389
                    tunnel: [w491] -> w393
                    tunnel: [w490] -> w392
                    tunnel: [w484] -> w376
                    tunnel: w369 -> [w483]
                    tunnel: w367 -> [w482]
                    tunnel: w366 -> [w481]
                    frame #0 {
                      # "calcute x_n+1"
                      n148 = Multiply(x=w412, y=w414) -> (x*y=w407:dbl)
                      n149 = Multiply(x=w412, y=w413) -> (x*y=w409:dbl)
                      n150 = Add(x=w407, y=w406) -> (x+y=w417:dbl)
                      n151 = Add(x=w409, y=w408) -> (x+y=w415:dbl)
                    }
                    frame #1 {
                      # "go to x_n+1"
                      n152 = invoke class="IntegratedStepperMotor" method="SetMoveAbsolutePosition"(reference=w425, "position"=w423) -> (reference out=w429:refnum<k24>, error out=w427:errorcluster)  [unwired: 2 in, 2 out]
                      n153 = invoke class="IntegratedStepperMotor" method="SetMoveAbsolutePosition"(reference=w424, "position"=w419) -> (reference out=w428:refnum<k24>, error out=w426:errorcluster)  [unwired: 2 in, 2 out]
                      n154 = Subtract(x=w423, y=w422) -> (x-y=w421:dbl)
                      n155 = Subtract(x=w419, y=w420) -> (x-y=w418:dbl)
                    }
                    frame #2 {
                      w433 = 250
                      n156 = Divide(x=5000, y=w433) -> (x/y=w435:dbl)
                      n157 = for {
                        N: w435 -> [_]
                        tunnel: w443 -> [w468]
                        tunnel: w442 -> [w467]
                        tunnel: w441 -> [w466]
                        tunnel: w440 -> [w465]
                        tunnel: w439 -> [w448]
                        tunnel: w438 -> [w449]
                        tunnel: [w449] -> w437
                        tunnel: [w448] -> w436
                        tunnel: w433 -> [w447]
                        stop <- w450 stop-if-true
                        w453 = 0.01 ("y")
                        w458 = 409600 ("y")
                        n158 = invoke class="IntegratedStepperMotor" method="GetPositionCounter"(reference=w468, error in=w466) -> (error out=w462:errorcluster, "GetPositionCounter"=w460:i32)  [unwired: 1 in, 1 out]
                        n159 = invoke class="IntegratedStepperMotor" method="GetPositionCounter"(reference=w467, error in=w465) -> (error out=w461:errorcluster, "GetPositionCounter"=w459:i32)  [unwired: 1 in, 1 out]
                        n160 = Wait (ms)(milliseconds to wait=w447) -> ()  [unwired: 1 out]
                        n161 = local read "stage-error"() -> (w464:errorcluster)
                        n162 = Merge Errors(w464, w462, w461) -> (w463:errorcluster)
                        n163 = Divide(x=w460, y=w458) -> (x/y=w446:dbl)
                        n164 = Divide(x=w459, y=w458) -> (x/y=w445:dbl)
                        n165 = local write "stage-error"(w463) -> ()
                        n166 = local write "bar_y_pos"(w445) -> ()
                        n167 = Subtract(x=w446, y=w449) -> (x-y=w457:dbl)
                        n168 = Subtract(x=w445, y=w448) -> (x-y=w456:dbl)
                        n169 = local write "bar_x_pos"(w446) -> ()
                        n170 = Absolute Value(x=w457) -> (abs(x)=w455:dbl)
                        n171 = Absolute Value(x=w456) -> (abs(x)=w454:dbl)
                        n172 = Less Or Equal?(x=w455, y=w453) -> (x <= y?=w452:bool)
                        n173 = Less Or Equal?(x=w454, y=w453) -> (x <= y?=w451:bool)
                        n174 = And(x=w452, y=w451) -> (x .and. y?=w450:bool)
                      }
                    }
                    frame #3 {
                      w475 = u16 2 items=["PD1", "PD2", "PD3"] ("Photodiode Select")
                      # "measure at x_n+1\nto get y_n+1"
                      n175 = local read "meter-error"() -> (w477:errorcluster)
                      n176 = local read "meter-visa"() -> (w478:refnum<visa-resource-name>)
                      n177 = local read "nSamples"() -> (w469:dbl)
                      n178 = call "meter_buffered - one channel.vi"("Samples"=w469, "error in"=w477, "Channel"=w475, "PD Range"=w473, "meter-VISA"=w478) -> ("error out"=w476:errorcluster, "avg"=w474:dbl)  [unwired: 3 in, 2 out]
                      n179 = local write "meter-error"(w476) -> ()
                      n180 = Subtract(x=w474, y=w473) -> (x-y=w472:dbl)
                    }
                    frame #4 {
                      # "calc gradient"
                      n181 = Equal To 0?(x=w482) -> (x = 0?=w486:bool)
                      n182 = Equal To 0?(x=w481) -> (x = 0?=w485:bool)
                      n183 = Divide(x=w483, y=w482) -> (x/y=w491:dbl)
                      n184 = Divide(x=w483, y=w481) -> (x/y=w490:dbl)
                      n185 = Or(x=w486, y=w485) -> (x .or. y?=w484:bool)
                    }
                  }
                }
              }
            }
          }
          frame #5 {
            # "Grid method alignment - runs only when initiated"
            n186 = And(x="auto-align-grid", y=FALSE) -> (x .and. y?=w493:bool)
            n187 = case shown="True" w493 {
              tunnel: w495 -> [_ w498]
              frame False {
              }
              frame True {
                n188 = Unbundle By Name(w498) -> ("PD X"=w497:refnum<k24>, "PD Y"=w496:refnum<k24>)
                n189 = local read "PD Values"() -> (w504:cluster{"PD1":dbl, "PD2":dbl, "PD3":dbl})
                n190 = Multiply(x="auto-delta", y=dbl[] [-2.0, -1.0, 0.0, 1.0, 2.0]) -> (x*y=w505:dbl[])
                n191 = local read "pd_x_pos"() -> (w502:dbl)
                n192 = local read "pd_y_pos"() -> (w501:dbl)
                n193 = Unbundle By Name(w504) -> ("PD3"=w503:dbl)
                n194 = Add(x=w502, y=w505) -> (x+y=w508:dbl[])
                n195 = Add(x=w501, y=w505) -> (x+y=w507:dbl[])
                n196 = for {
                  tunnel: w508 -> [w525] mode=indexing
                  tunnel: w507 -> [w526]
                  tunnel: [w524] -> w515 mode=indexing
                  tunnel: [w523] -> w516 mode=indexing
                  tunnel: [w522] -> w510 mode=indexing
                  tunnel: w497 -> [w521]
                  tunnel: w496 -> [w520]
                  tunnel: w503 -> [w519]
                  n197 = for {
                    tunnel: w526 -> [w544] mode=indexing
                    tunnel: w525 -> [w543]
                    tunnel: [w542] -> w523 mode=indexing
                    tunnel: [w541] -> w524 mode=indexing
                    tunnel: [w540] -> w522 mode=indexing
                    tunnel: w521 -> [w535]
                    tunnel: w520 -> [w534]
                    tunnel: w519 -> [w529]
                    n198 = flat-sequence {
                      tunnel: w544 -> [w550]
                      tunnel: w543 -> [w552]
                      tunnel: [w552] -> w539
                      tunnel: [w550] -> w537
                      tunnel: w535 -> [w553]
                      tunnel: w534 -> [w551]
                      tunnel: [w549] -> w533
                      tunnel: [w548] -> w532
                      tunnel: [w547] -> w531
                      tunnel: [w546] -> w530
                      tunnel: w529 -> [w545]
                      tunnel: [w545] -> w527
                      tunnel: w539 -> [w562]
                      tunnel: [w562] -> w538
                      tunnel: w537 -> [w563]
                      tunnel: [w563] -> w536
                      tunnel: w533 -> [w561]
                      tunnel: w532 -> [w560]
                      tunnel: w531 -> [w559]
                      tunnel: w530 -> [w558]
                      tunnel: [w554] -> w528
                      tunnel: w527 -> [w554]
                      tunnel: [w596] -> w542
                      tunnel: w538 -> [w596]
                      tunnel: [w595] -> w541
                      tunnel: w536 -> [w595]
                      tunnel: [w594] -> w540
                      tunnel: w528 -> [w588]
                      frame #0 {
                        # "Move to x, y"
                        n199 = invoke class="IntegratedStepperMotor" method="SetMoveAbsolutePosition"(reference=w553, "position"=w552) -> (reference out=w549:refnum<k24>, error out=w548:errorcluster)  [unwired: 2 in, 2 out]
                        n200 = invoke class="IntegratedStepperMotor" method="SetMoveAbsolutePosition"(reference=w551, "position"=w550) -> (reference out=w547:refnum<k24>, error out=w546:errorcluster)  [unwired: 2 in, 2 out]
                      }
                      frame #1 {
                        w556 = 250
                        # "verify at x, y"
                        n201 = Divide(x=5000, y=w556) -> (x/y=w557:dbl)
                        n202 = for {
                          N: w557 -> [_]
                          tunnel: w561 -> [w587]
                          tunnel: w559 -> [w586]
                          tunnel: w560 -> [w585]
                          tunnel: w558 -> [w584]
                          tunnel: w563 -> [w567]
                          tunnel: w562 -> [w568]
                          tunnel: w556 -> [w566]
                          stop <- w569 stop-if-true
                          w572 = 0.01 ("y")
                          w577 = 409600 ("y")
                          n203 = invoke class="IntegratedStepperMotor" method="GetPositionCounter"(reference=w587, error in=w585) -> (error out=w581:errorcluster, "GetPositionCounter"=w579:i32)  [unwired: 1 in, 1 out]
                          n204 = invoke class="IntegratedStepperMotor" method="GetPositionCounter"(reference=w586, error in=w584) -> (error out=w580:errorcluster, "GetPositionCounter"=w578:i32)  [unwired: 1 in, 1 out]
                          n205 = Wait (ms)(milliseconds to wait=w566) -> ()  [unwired: 1 out]
                          n206 = local read "stage-error"() -> (w583:errorcluster)
                          n207 = Merge Errors(w583, w581, w580) -> (w582:errorcluster)
                          n208 = Divide(x=w579, y=w577) -> (x/y=w565:dbl)
                          n209 = Divide(x=w578, y=w577) -> (x/y=w564:dbl)
                          n210 = local write "bar_y_pos"(w564) -> ()
                          n211 = Subtract(x=w565, y=w568) -> (x-y=w576:dbl)
                          n212 = local write "bar_x_pos"(w565) -> ()
                          n213 = local write "stage-error"(w582) -> ()
                          n214 = Subtract(x=w564, y=w567) -> (x-y=w575:dbl)
                          n215 = Absolute Value(x=w576) -> (abs(x)=w574:dbl)
                          n216 = Absolute Value(x=w575) -> (abs(x)=w573:dbl)
                          n217 = Less Or Equal?(x=w574, y=w572) -> (x <= y?=w571:bool)
                          n218 = Less Or Equal?(x=w573, y=w572) -> (x <= y?=w570:bool)
                          n219 = And(x=w571, y=w570) -> (x .and. y?=w569:bool)
                        }
                      }
                      frame #2 {
                        w590 = u16 2 items=["PD1", "PD2", "PD3"] ("Photodiode Select")
                        # "DAQ"
                        n220 = local read "meter-visa"() -> (w593:refnum<visa-resource-name>)
                        n221 = local read "meter-error"() -> (w592:errorcluster)
                        n222 = call "meter_buffered - one channel.vi"("Samples"=u32 50 ("preDAQ  wait ms"), "error in"=w592, "Channel"=w590, "PD Range"=w588, "meter-VISA"=w593) -> ("error out"=w591:errorcluster, "avg"=w594:dbl)  [unwired: 3 in, 2 out]
                        n223 = local write "meter-error"(w591) -> ()
                      }
                    }
                  }
                }
                n224 = Array Max & Min(array=w510) -> (max value=→"max value":dbl, max index (indices)=w512:i32[])  [unwired: 2 out]
                "max indexes" <- w512
                n225 = Index Array(array=w512, index #1=0 ("index"), index #2=1 ("index")) -> (element #1=w500:i32, element #2=w499:i32)
                n226 = Index Array(array=w516, index (row)=w500, index (col)=w499) -> (element=→"xOut":dbl)
                n227 = Index Array(array=w515, index (row)=w500, index (col)=w499) -> (element=→"yOut":dbl)
              }
            }
          }
        }
        n228 = Subtract(x=w89, y=w88) -> (x-y=→"loop-rate":u32)
        n229 = Wait (ms)(milliseconds to wait=u32 5) -> ()  [unwired: 1 out]
        n230 = property on="start-msg" class="Str"("Visible"=FALSE) -> ()  [unwired: 2 in, 2 out]
        n231 = Get Date/Time In Seconds() -> (seconds since 1Jan1904=w83:timestamp)
        n232 = Format Date/Time String(time format string (%c)="%Y-%m-%d %H:%M:%S", seconds (now)=w83) -> (date/time string=→"Current Time:":string)  [unwired: 1 in]
      }
      n233 = invoke class="LongTravelStageControl" method="CloseDevice"(reference=w78) -> (error out=w55:errorcluster)  [unwired: 2 in, 2 out]
      n234 = invoke class="LongTravelStageControl" method="CloseDevice"(reference=w65) -> (error out=w54:errorcluster)  [unwired: 2 in, 2 out]
      n235 = invoke class="LongTravelStageControl" method="CloseDevice"(reference=w66) -> (error out=w53:errorcluster)  [unwired: 2 in, 2 out]
      n236 = invoke class="LongTravelStageControl" method="CloseDevice"(reference=w67) -> (error out=w52:errorcluster)  [unwired: 2 in, 2 out]
      n237 = invoke class="BenchtopStepperControl" method="CloseDevice"(reference=w59) -> (error out=w51:errorcluster)  [unwired: 2 in, 2 out]
      n238 = invoke class="BenchtopStepperControl" method="CloseDevice"(reference=w56) -> (error out=w50:errorcluster)  [unwired: 2 in, 2 out]
      n239 = local read "stage-error"() -> (w33:errorcluster)
      n240 = Merge Errors(w33, w55, w54, w53, w52, w51, w50) -> (w32:errorcluster)
      n241 = local write "stage-error"(w32) -> ()
    }
    frame #3 {
      # "Close connection to meter"
      n242 = local read "meter-error"() -> (w598:errorcluster)
      n243 = local read "meter-visa"() -> (w597:refnum<visa-resource-name>)
      n244 = call <instrlib>:"Close.vi"("error in (no error)"=w598, "VISA resource name"=w597) -> ("error out"=w599:errorcluster)  [unwired: 9 in]
      n245 = local write "meter-error"(w599) -> ()
    }
    frame #4 {
      # "Section deletes log file if nothing is written to it\nto prevent just a ton of empty files during development"
      n246 = local read "log-path"() -> (w601:path)
      n247 = local read "log-error"() -> (w606:errorcluster)
      n248 = Open/Create/Replace File(file path (use dialog)=w601, error in=w606) -> (refnum out=w611:refnum<file>, error out=w610:errorcluster)  [unwired: 4 in, 1 out]
      n249 = Read from Text File(file (use dialog)=w611, error in=w610) -> (refnum out=w608:refnum<file>, text=w609:string, error out=w607:errorcluster)  [unwired: 2 in, 1 out]
      n250 = Equal?(x="T, PD1, PD2, PD3, Bar Note\n" ("Display"), y=w609) -> (x = y?=w605:bool)
      n251 = Close File(refnum=w608, error in=w607) -> (path=w604:path, error out=w603:errorcluster)
      n252 = case shown="False" w605 {
        tunnel: w604 -> [_ w615]
        tunnel: w603 -> [w612 w614]
        tunnel: [w612 w613] -> w602
        frame False {
        }
        frame True {
          n253 = Delete(path (use dialog)=w615, error in=w614) -> (error out=w613:errorcluster)  [unwired: 3 in, 2 out]
        }
      }
      n254 = local write "log-error"(w602) -> ()
    }
  }
